vi "Generic_NPT.vi"() -> ()   [LabVIEW 2016]
panel:
  out "Graph":u16[](graph)
  in  "stop":bool
  # "Connect proper signal to channel A before starting acquisition\n(e.g. 1Vpp 1kHz sine wave)"
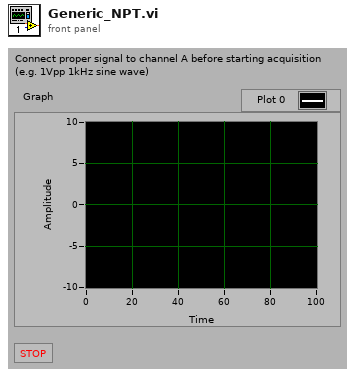
[diagram p1: front panel]
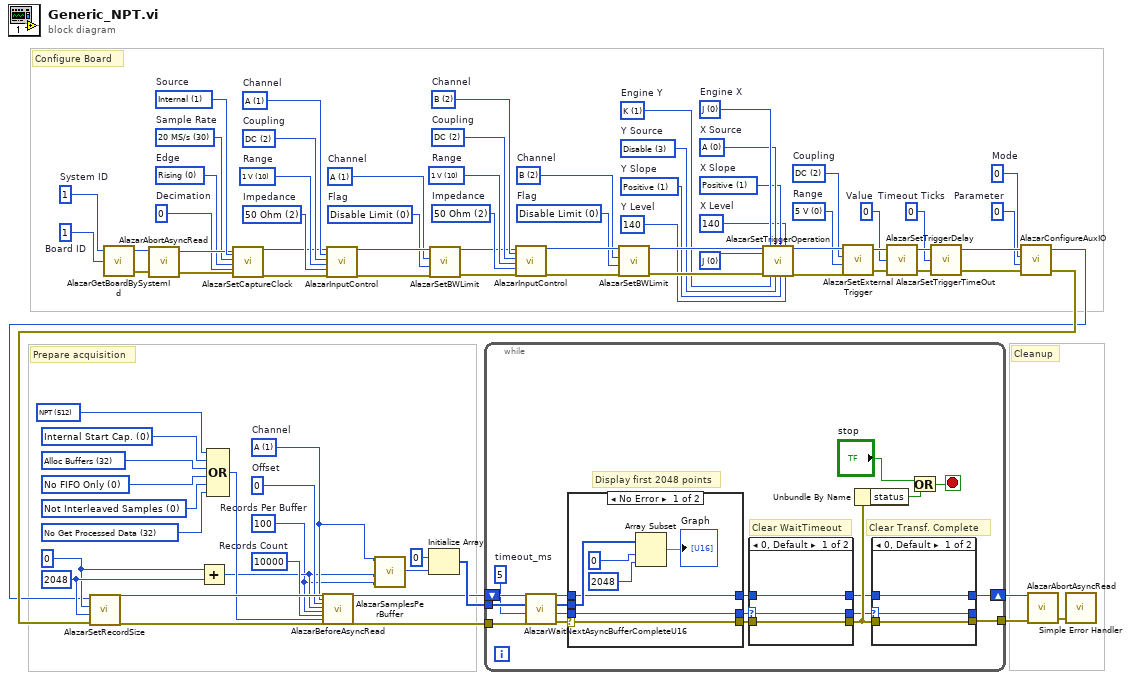
[diagram p0: block diagram]
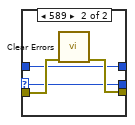
[diagram p2: hidden frame]
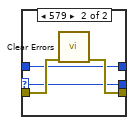
[diagram p3: hidden frame]
diagram:
  w14 = u32 10000  # Records Count
  w2 = u32 100  # Records Per Buffer
  w15 = u32 0  # Offset
  w4 = u32 1 items=["A"=1, "B"=2, "A + B"=3, "C"=4, "A + C"=5, "A + B"=6, "D"=8, "A + D"=9, "B + D"=10, "C + D"=12, "A + B + C + D"=15]  # Channel
  w20 = u32 2048 ("Post-trigger Samples")
  w19 = u32 0 ("Pre-trigger Samples")
  w26 = u32 32 items=["No Get Processed Data"=32, "Get Processed Data"=8192]
  w25 = u32 0 items=["Not Interleaved Samples"=0, "Interleave Samples"=4096]
  w21 = u32 0 items=["No FIFO Only"=0, "FIFO Only"=2048]
  w24 = u32 32 items=["Alloc Buffers"=32]
  w23 = u32 0 items=["Internal Start Cap.", "External Start Cap."]
  w22 = u32 512 items=["Traditional"=0, "NPT"=512, "Continuous"=256, "Triggered Streaming"=1024]
  w56 = u32 0 items=["Disable Limit", "Enable Limit"]  # Flag
  w55 = u32 2 items=["A"=1, "B"=2, "C"=4, "D"=8]  # Channel
  w59 = u32 2 items=["1 MOhm"=1, "50 Ohm"=2]  # Impedance
  w53 = u32 10 items=["20 mV"=1, "40 mV"=2, "50 mV"=3, "80 mV"=4, "100 mV"=5, "200 mV"=6, "400 mV"=7, "500 mV"=8, "800 mV"=9, "1 V"=10, "1.25 V"=33, "2 V"=11, "4 V"=12, "5 V"=13, "8 V"=14, "10 V"=15, "20 V"=16]  # Range
  w60 = u32 2 items=["AC"=1, "DC"=2]  # Coupling
  w61 = u8 2 items=["A"=1, "B"=2, "C"=4, "D"=8]  # Channel
  w29 = u32 0  # Parameter
  w28 = u32 0  # Mode
  w27 = u32 0  # Timeout Ticks
  w34 = u32 0  # Value
  w38 = u32 0 items=["5 V", "1 V", "TTL"]  # Range
  w37 = u32 2 items=["AC"=1, "DC"=2]  # Coupling
  w41 = u32 140  # Y Level
  w42 = u32 1 items=["Positive"=1, "Negative"=2]  # Y Slope
  w43 = u32 3 items=["A", "B", "External", "Disable", "C", "D"]  # Y Source
  w45 = u32 140  # X Level
  w46 = u32 1 items=["Positive"=1, "Negative"=2]  # X Slope
  w47 = u32 0 items=["A", "B", "External", "Disable", "C", "D"]  # X Source
  w44 = u32 1 items=["J", "K"]  # Engine Y
  w48 = u32 0 items=["J", "K"]  # Engine X
  w49 = u32 0 items=["J", "K", "J OR K", "J AND K", "J XOR K", "J AND NOT K", "NOT J AND K"] ("Op.")
  w63 = u32 0 items=["Disable Limit", "Enable Limit"]  # Flag
  w62 = u32 1 items=["A"=1, "B"=2, "C"=4, "D"=8]  # Channel
  w68 = u32 2 items=["1 MOhm"=1, "50 Ohm"=2]  # Impedance
  w69 = u32 10 items=["20 mV"=1, "40 mV"=2, "50 mV"=3, "80 mV"=4, "100 mV"=5, "200 mV"=6, "400 mV"=7, "500 mV"=8, "800 mV"=9, "1 V"=10, "1.25 V"=33, "2 V"=11, "4 V"=12, "5 V"=13, "8 V"=14, "10 V"=15, "20 V"=16]  # Range
  w70 = u32 2 items=["AC"=1, "DC"=2]  # Coupling
  w71 = u8 1 items=["A"=1, "B"=2, "C"=4, "D"=8]  # Channel
  w73 = u32 0  # Decimation
  w74 = u32 0 items=["Rising", "Falling"]  # Edge
  w75 = u32 30 items=["1 kS/s"=1, "2 kS/s"=2, "5 kS/s"=4, "10 kS/s"=8, "20 kS/s"=10, "50 kS/s"=12, "100 kS/s"=14, "200 kS/s"=16, "500 kS/s"=18, "1 MS/s"=20, "2 MS/s"=24, "5 MS/s"=26, "10 MS/s"=28, "20 MS/s"=30, "25 MS/s"=33, "50 MS/s"=34, "100 MS/s"=36, "125 MS/s"=37, "160 MS/s"=38, "180 MS/s"=39, "250 MS/s"=43, "500 MS/s"=48, "800 MS/s"=50, "1000 MS/s"=53, "1200 MS/s"=55, "1500 MS/s"=58, "1800 MS/s"=61, "USER_DEF"=0]  # Sample Rate
  w77 = u32 1 items=["Internal"=1, "Fast External"=2, "Medium External"=3, "Slow External"=4, "External AC"=5, "External DC"=6, "External 10MHz"=7]  # Source
  w81 = u32 1  # Board ID
  w80 = u32 1  # System ID
  # "Cleanup"
  # "Prepare acquisition"
  # "Configure Board"
  n1 = call "AlazarGetBoardBySystemId.vi"("Board ID"=w81, "System ID"=w80) -> ("error out"=w78:errorcluster, "Handle"=w79:u64)  [unwired: 1 in, 1 out]
  n2 = call "AlazarAbortAsyncRead.vi"("Handle"=w79, "error in (no error)"=w78) -> ("Handle"=w76:u64, "error out"=w72:errorcluster)  [unwired: 1 out]
  n3 = Add(x=w19, y=w20) -> (x+y=w3:u32)
  n4 = Compound Arithmetic op=OR(w22, w23, w24, w21, w25, w26) -> (w16:u32)
  n5 = call "AlazarSetCaptureClock.vi"("Handle"=w76, "Source"=w77, "Sample Rate"=w75, "Edge"=w74, "Decimation"=w73, "error in (no error)"=w72) -> ("Handle"=w67:u64, "error out"=w66:errorcluster)  [unwired: 11 in, 1 out]
  n6 = call "AlazarInputControl.vi"("Handle"=w67, "Channel"=w71, "Coupling"=w70, "Range"=w69, "Impedance"=w68, "error in (no error)"=w66) -> ("Handle"=w65:u64, "error out"=w64:errorcluster)  [unwired: 11 in, 1 out]
  n7 = call "AlazarSamplesPerBuffer.vi"("Records Per Buffer"=w2, "Samples Per Record"=w3, "Channel Mask"=w4) -> ("Samples Per Buffer"=w1:u32)  [unwired: 1 in]
  n8 = Initialize Array(u16 0, w1) -> (w12:u16[])
  n9 = call "AlazarSetBWLimit.vi"("error in (no error)"=w64, "Flag"=w63, "Channel"=w62, "Handle"=w65) -> ("error out"=w54:errorcluster, "Handle"=w52:u64)  [unwired: 1 out]
  n10 = call "AlazarInputControl.vi"("Handle"=w52, "Channel"=w61, "Coupling"=w60, "Range"=w53, "Impedance"=w59, "error in (no error)"=w54) -> ("Handle"=w58:u64, "error out"=w57:errorcluster)  [unwired: 11 in, 1 out]
  n11 = call "AlazarSetBWLimit.vi"("error in (no error)"=w57, "Flag"=w56, "Channel"=w55, "Handle"=w58) -> ("error out"=w50:errorcluster, "Handle"=w51:u64)  [unwired: 1 out]
  n12 = call "AlazarSetTriggerOperation.vi"("Handle"=w51, "Trigger Operation"=w49, "error in (no error)"=w50, "Trigger Engine 1"=w48, "Trigger Engine 2"=w44, "Source 1"=w47, "Source 2"=w43, "Slope 1"=w46, "Slope 2"=w42, "Level 1"=w45, "Level 2"=w41) -> ("Handle"=w40:u64, "error out"=w39:errorcluster)  [unwired: 6 in, 1 out]
  n13 = call "AlazarSetExternalTrigger.vi"("error in (no error)"=w39, "Range ID"=w38, "Coupling ID"=w37, "Handle"=w40) -> ("error out"=w35:errorcluster, "Handle"=w36:u64)  [unwired: 1 out]
  n14 = call "AlazarSetTriggerDelay.vi"("error in (no error)"=w35, "Delay"=w34, "Handle"=w36) -> ("error out"=w32:errorcluster, "Handle"=w33:u64)  [unwired: 1 out]
  n15 = call "AlazarSetTriggerTimeOut.vi"("error in (no error)"=w32, "Timeout Ticks"=w27, "Handle"=w33) -> ("error out"=w30:errorcluster, "Handle"=w31:u64)  [unwired: 1 out]
  n16 = call "AlazarConfigureAuxIO.vi"("error in (no error)"=w30, "Parameter"=w29, "Mode"=w28, "Handle"=w31) -> ("error out"=w6:errorcluster, "Handle"=w5:u64)  [unwired: 1 out]
  n17 = call "AlazarSetRecordSize.vi"("error in (no error)"=w6, "Post-trigger Samples"=w20, "Pre-trigger Samples"=w19, "Handle"=w5) -> ("error out"=w17:errorcluster, "Handle"=w18:u64)  [unwired: 1 out]
  n18 = call "AlazarBeforeAsyncRead.vi"("Handle"=w18, "Channel Select"=w4, "Transfer Offset"=w15, "Transfer Length"=w3, "Records Per Buffer"=w2, "Records Per Acquisition"=w14, "Flags"=w16, "error in (no error)"=w17) -> ("Handle"=w11:u64, "error out"=w10:errorcluster)  [unwired: 17 in, 1 out]
  n19 = while {
    tunnel: w12 -> [w100]
    tunnel: w10 -> [w97]
    tunnel: [w82] -> w7
    shift-right: [w83] -> w8
    shift-left: w11 -> [w99]
    stop <- w86 stop-if-true
    w98 = u32 5  # timeout_ms
    # "Clear Transf. Complete"
    # "Clear WaitTimeout"
    # "Display first 2048 points"
    n20 = call "AlazarWaitNextAsyncBufferCompleteU16.vi"("error in (no error)"=w97, "Timeout (ms)"=w98, "Buffer"=w100, "Handle"=w99) -> ("error out"=w96:errorcluster, "Return Code"=w95:u32, "Buffer"=w90:u16[], "Handle"=w92:u64)
    n21 = case shown="No Error" w96 {
      selector: w96 -> [w115 w123]
      tunnel: w95 -> [w117 w124]
      tunnel: [w117 w124] -> w94
      tunnel: [w115 w123] -> w93
      tunnel: [w116 w122] -> w91
      tunnel: w92 -> [w116 w122]
      tunnel: w90 -> [w120 _]
      frame No Error {
        n22 = Array Subset(array=w120, index=0, length=2048) -> (→"Graph":u16[])
      }
      frame Error {
      }
    }
    n23 = case shown="0, Default" w94 {
      selector: w94 -> [w109 w111]
      tunnel: w93 -> [w108 w114]
      tunnel: [w108 w113] -> w89
      tunnel: [w110 w112] -> w88
      tunnel: w91 -> [w110 w112]
      tunnel: [w109 w111] -> w87
      frame 0, Default {
      }
      frame 579 {
        n24 = call <vilib>:"Clear Errors.vi"("error in (no error)"=w114) -> ("error out"=w113:errorcluster)  [unwired: 5 in, 1 out]
      }
    }
    n25 = Unbundle By Name(w89) -> ("status"=w84:bool)
    n26 = case shown="0, Default" w87 {
      selector: w87 -> [w102 w104]
      tunnel: w89 -> [w101 w107]
      tunnel: [w101 w106] -> w82
      tunnel: [w103 w105] -> w83
      tunnel: w88 -> [w103 w105]
      tunnel: [w102 w104] -> _
      frame 0, Default {
      }
      frame 589 {
        n27 = call <vilib>:"Clear Errors.vi"("error in (no error)"=w107) -> ("error out"=w106:errorcluster)  [unwired: 5 in, 1 out]
      }
    }
    n28 = Or(x="stop", y=w84) -> (x .or. y?=w86:bool)
  }
  n29 = call "AlazarAbortAsyncRead.vi"("Handle"=w8, "error in (no error)"=w7) -> ("error out"=w9:errorcluster)  [unwired: 2 out]
  n30 = call <vilib>:"Simple Error Handler.vi"("error in (no error)"=w9) -> ()  [unwired: 4 in, 5 out]
